vi "getCounterPosition.vi"(0 "PMX4CXSAController in":refnum<class "PMX4CXSAController.lvclass">, 2 "type (nc)":T2, 5 "error in (no error)":errorcluster) -> (14 "PMX4CXSAController out":refnum<class "PMX4CXSAController.lvclass">, 16 "counter_vals (nc)":T1, 19 "error out":errorcluster)   [LabVIEW 2020, in "classes.lvlib" / "PMX4CXSAController.lvclass"]
doc: "Produced By:\n\n<B>Kod Integrations, LLC</B>\n4835 Marianne Drive\nMount Airy, MD 21771\nhttp://www.kodintegrations.com\nemail: info@kodintegrations.com\nphone: (240) 687-1288"
uses:
  PMX4CXSAController.lvclass
  C:/GEECS/Developers Version/source/Device Drivers/Newmark-NSC-A/Arcus Driver 3.0.0/ArcusUsbComm/classes/Controller/_Controller.lvclass
  counter_type.ctl
  counter_values.ctl
  _Controller.lvclass/_Controller.ctl
  _Controller.lvclass
  common.lvlib
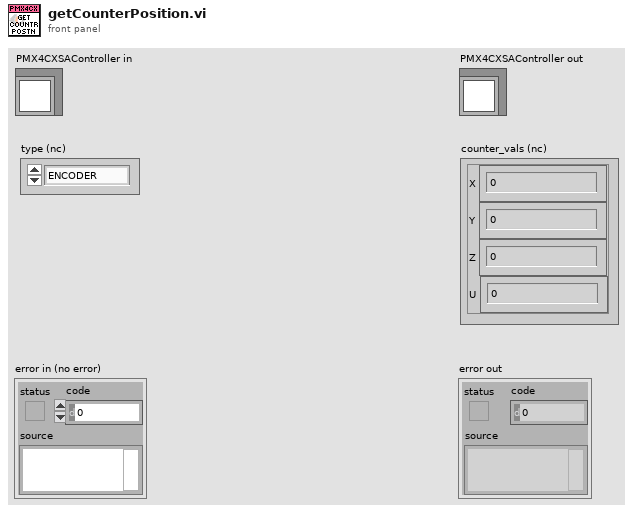
[diagram p1: front panel]
types:
  T1 = typedef "common.lvlib/counter_values.ctl" = cluster{"X":i32, "Y":i32, "Z":i32, "U":i32}
  T2 = typedef "common.lvlib/counter_type.ctl" = enum16{"ENCODER", "PULSE"}
  T3 = typedef "common.lvlib/models.ctl" = enum16{"<unrecognized>", "ACE-SDC", "ACE-SDE", "ACE-SXC", "ACE-SXE", "DMX-CAN", "DMX-J-SA", "DMX-K-SA", "DMX-UMD", "PMX-2ED-SA", "PMX-2EX-SA", "PMX-4CX-SA", "PMX-4EX-SA"}
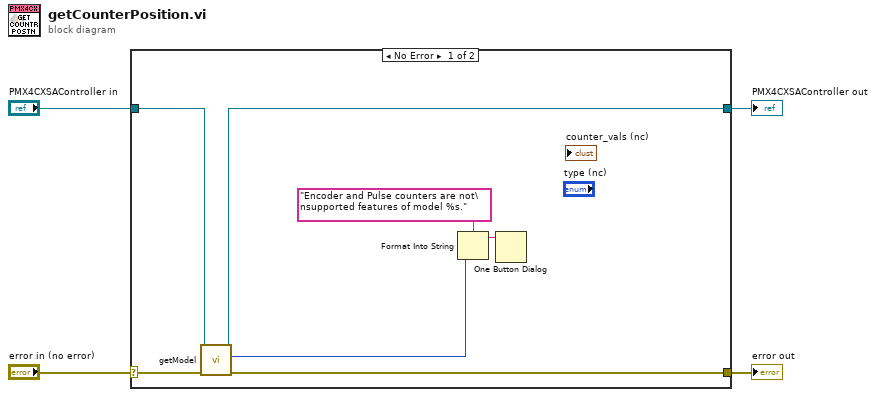
[diagram p0: block diagram]
diagram:
  n1 = case shown="No Error" "error in (no error)" {
    selector: "error in (no error)" -> [w11 w13]
    tunnel: [w10 w13] -> w3
    tunnel: [w6 w12] -> w1
    tunnel: "PMX4CXSAController in" -> [w7 w12]
    frame No Error {
      n2 = call "getModel.vi"("error in (no error)"=w11, "reference (in)"=w7) -> ("error out"=w10:errorcluster, "model"=w8:T3, "reference (out)"=w6:refnum<class "PMX4CXSAController.lvclass">)  [unwired: 7 in]
      n3 = Format Into String(format string="Encoder and Pulse counters are not\nsupported features of model %s.", w8) -> (resulting string=w5:string)  [unwired: 2 in, 1 out]
      n4 = One Button Dialog(message=w5) -> ()  [unwired: 1 in, 1 out]
    }
    frame Error {
    }
  }
  "error out" <- w3
  "PMX4CXSAController out" <- w1
